vi "主VI 2.vi"() -> ()   [LabVIEW 2010]
panel:
  out "Array 2":i32[](array[numeric])
  out "Array":i32[](array[numeric])
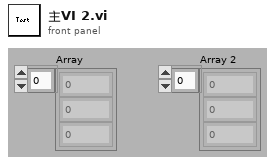
[diagram p1: front panel]
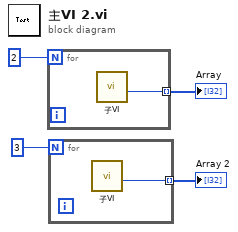
[diagram p0: block diagram]
diagram:
  n1 = for {
    N: 2 -> [_]
    tunnel: [w5] -> w4 mode=indexing
    n2 = call "子VI.vi"() -> ("output"=w5:i32)  [unwired: 11 in]
  }
  "Array" <- w4
  n3 = for {
    N: 3 -> [_]
    tunnel: [w6] -> w3 mode=indexing
    n4 = call "子VI.vi"() -> ("output"=w6:i32)  [unwired: 11 in]
  }
  "Array 2" <- w3
